vi "Batch Command.vi"() -> ()   [LabVIEW 2018]
panel:
  out "cmd sent":string
  out "test ready":string
  out "status":string
  out "mech":string
  out "state":u8
  out "S4ICS cmd":string
  out "LOG time":timestamp format="%<%H:%M:%S%3u\n%Y/%m/%d>T"
  in  "batch file":string="WPROT" caption="Batch File Name"
  in  "allin":T1={"s4icsIP"="localhost", "s4icsPort"=54165, "mech name"="", "cmd"=[], "log"=refnum} {"s4icsPort" min=1025 step=1}
  in  "stop":bool
  # "S4ICS Batch Command"
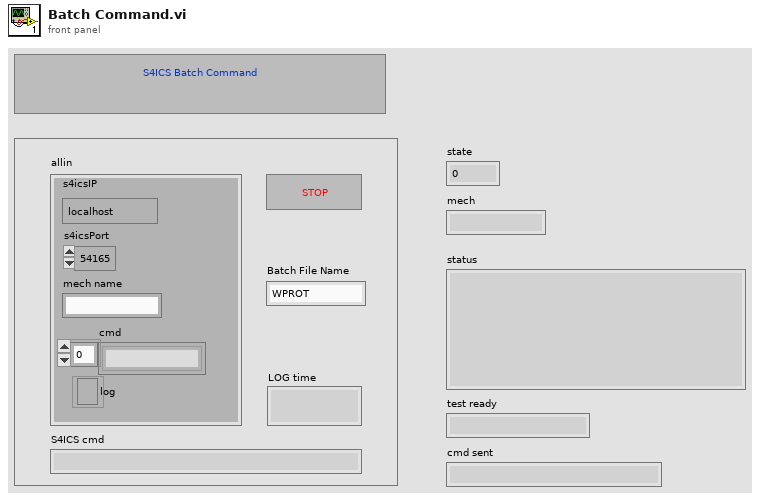
[diagram p1: front panel]
types:
  T1 = cluster{"s4icsIP":string, "s4icsPort":u16, "mech name":string, "cmd":string[], "log":refnum<file>}
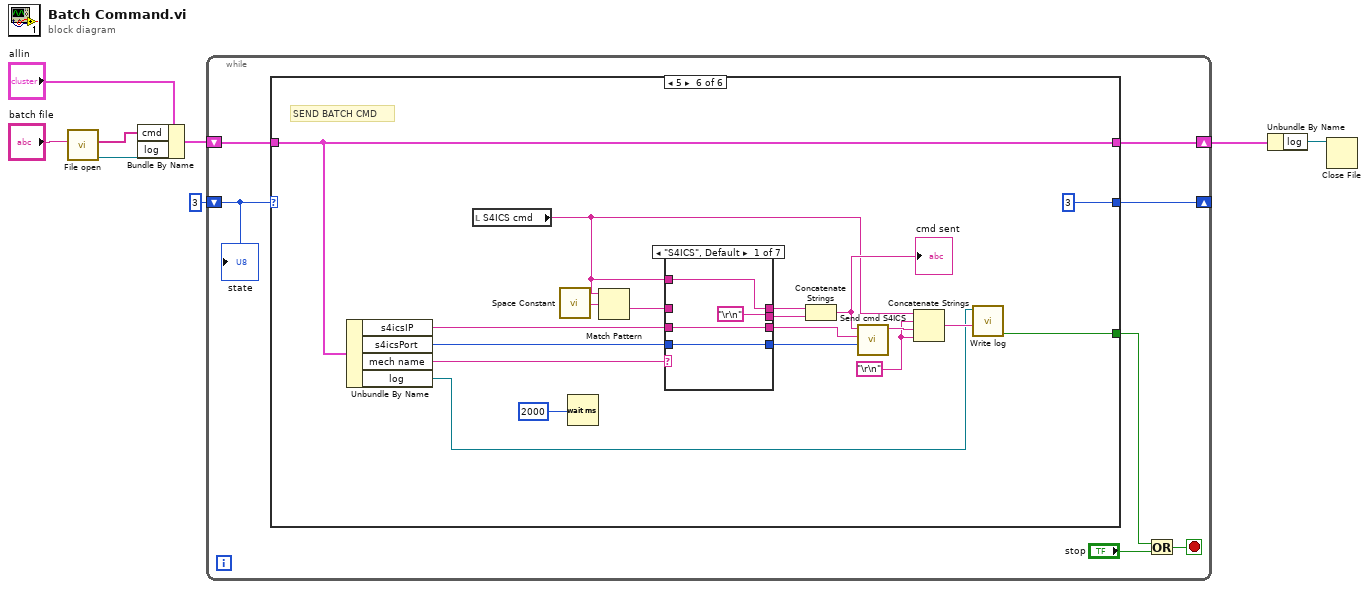
[diagram p0: block diagram]
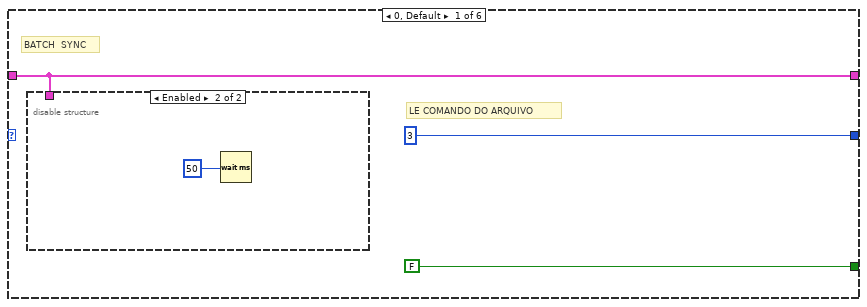
[diagram p2: hidden frame]
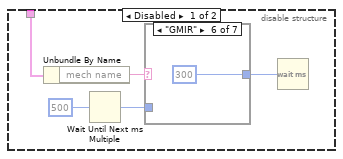
[diagram p3: hidden frame]
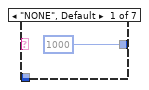
[diagram p4: hidden frame]
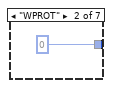
[diagram p5: hidden frame]
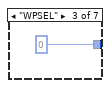
[diagram p6: hidden frame]
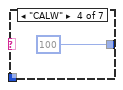
[diagram p7: hidden frame]
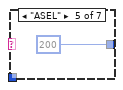
[diagram p8: hidden frame]
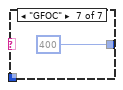
[diagram p9: hidden frame]
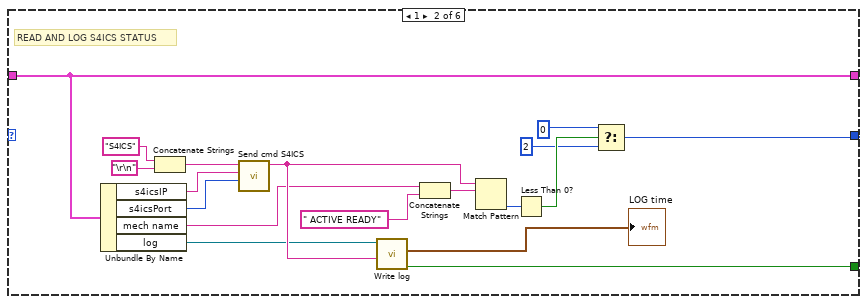
[diagram p10: hidden frame]
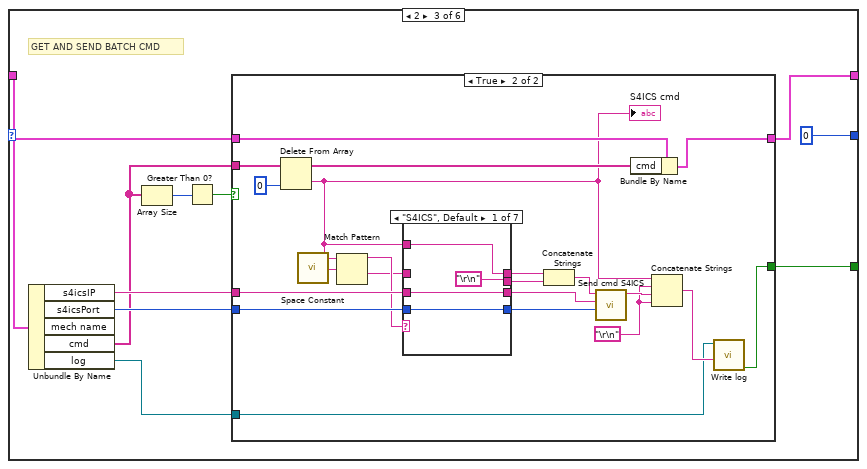
[diagram p11: hidden frame]
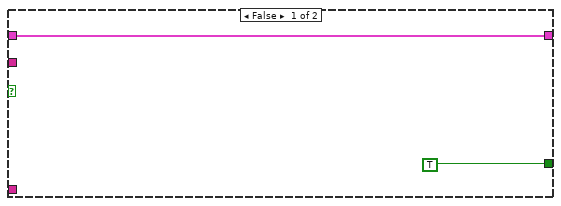
[diagram p12: hidden frame]
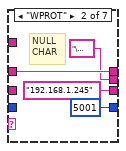
[diagram p13: hidden frame]
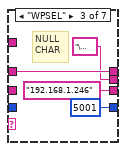
[diagram p14: hidden frame]
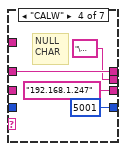
[diagram p15: hidden frame]
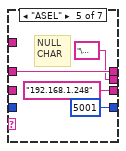
[diagram p16: hidden frame]
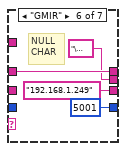
[diagram p17: hidden frame]
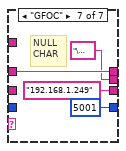
[diagram p18: hidden frame]
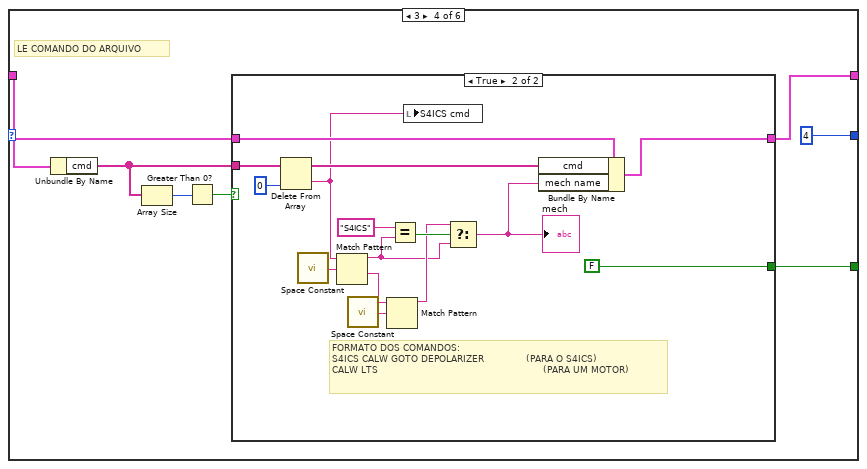
[diagram p19: hidden frame]
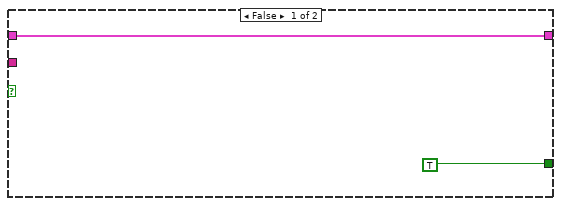
[diagram p20: hidden frame]
diagram:
  n1 = call "File open.vi"("file name"="batch file") -> ("log"=w5:refnum<file>, "cmd"=w4:string[])  [unwired: 9 in]
  n2 = Bundle By Name(cluster="allin", "cmd"=w4, "log"=w5) -> (w6:T1)
  n3 = while {
    shift-right: [w14] -> _
    shift-left: u8 3 -> [w15]
    shift-right: [w12] -> w2
    shift-left: w6 -> [w13]
    stop <- w10 stop-if-true
    n4 = case shown="5" w15 {
      tunnel: [u8 3 ("x+1") w40 u8 0 ("x+1") u8 4 ("x+1") w144 u8 3 ("x+1")] -> w14
      tunnel: w13 -> [w16 w42 w55 w115 w146 w170]
      tunnel: [w16 w42 w52 w112 w146 w170] -> w12
      tunnel: [FALSE w37 w54 w114 w141 w158] -> w9
      frame 0, Default {
        # "LE COMANDO DO ARQUIVO"
        # "BATCH  SYNC"
        n5 = disable-structure shown="Enabled" {
          disable-tunnel: w16 -> [w22 _]
          frame Disabled {
            n6 = Unbundle By Name(w22) -> ("mech name"=w21:string)
            n7 = Wait Until Next ms Multiple(millisecond multiple=u32 500) -> (millisecond timer value=w19:u32)
            n8 = case shown="\"GMIR\"" w21 {
              tunnel: [u32 1000 ("millisecond multiple") u32 0 ("millisecond multiple") u32 0 ("millisecond multiple") u32 100 ("millisecond multiple") u32 200 ("millisecond multiple") u32 300 ("millisecond multiple") u32 400 ("millisecond multiple")] -> w23
              tunnel: w19 -> [_ _ _ _ _ _ _]
              frame "NONE", Default {
              }
              frame "WPROT" {
              }
              frame "WPSEL" {
              }
              frame "CALW" {
              }
              frame "ASEL" {
              }
              frame "GMIR" {
              }
              frame "GFOC" {
              }
            }
            n9 = Wait (ms)(milliseconds to wait=w23) -> ()  [unwired: 1 out]
          }
          frame Enabled {
            n10 = Wait (ms)(milliseconds to wait=u32 50 ("millisecond multiple")) -> ()  [unwired: 1 out]
          }
        }
      }
      frame 1 {
        # "READ AND LOG S4ICS STATUS"
        n11 = Unbundle By Name(w42) -> ("s4icsIP"=w47:string, "s4icsPort"=w46:u16, "mech name"=w34:string, "log"=w36:refnum<file>)
        n12 = Concatenate Strings("S4ICS", "\r\n") -> (w45:string)
        n13 = call "Send cmd S4ICS.vi"("port"=w46, "address"=w47, "data in"=w45) -> ("data out"=w38:string)  [unwired: 7 in, 1 out]
        n14 = call "Write log.vi"("text"=w38, "log file"=w36) -> ("status"=w37:bool, "current time"=→"LOG time":timestamp)  [unwired: 8 in]
        n15 = Concatenate Strings(w34, " ACTIVE READY") -> (w35:string)
        n16 = Match Pattern(string=w38, regular expression=w35) -> (offset past match=w44:i32)  [unwired: 1 in, 3 out]
        n17 = Less Than 0?(x=w44) -> (x < 0?=w41:bool)
        n18 = Select(t=u8 0 ("f"), s=w41, f=u8 2) -> (s? t:f=w40:u8)
      }
      frame 2 {
        # "GET AND SEND BATCH CMD"
        n19 = Unbundle By Name(w55) -> ("s4icsIP"=w59:string, "s4icsPort"=w58:u16, "cmd"=w51:string[], "log"=w50:refnum<file>)  [unwired: 1 out]
        n20 = Array Size(array=w51) -> (size(s)=w57:i32)
        n21 = Greater Than 0?(x=w57) -> (x > 0?=w56:bool)
        n22 = case shown="True" w56 {
          tunnel: w59 -> [_ w72]
          tunnel: w58 -> [_ w71]
          tunnel: w51 -> [_ w82]
          tunnel: w55 -> [w61 w81]
          tunnel: [w61 w80] -> w52
          tunnel: [TRUE w76] -> w54
          tunnel: w50 -> [_ w73]
          frame False {
          }
          frame True {
            w74 = "\r\n"
            n23 = Delete From Array(array=w82, index=0) -> (deleted portion=w64:string, array with subset deleted=w77:string[])  [unwired: 1 in]
            "S4ICS cmd" <- w64
            n24 = call <vilib>:"Space Constant.vi"() -> ("String"=w67:string)
            n25 = Match Pattern(string=w64, regular expression=w67) -> (before substring=w66:string, after substring=w65:string)  [unwired: 1 in, 2 out]
            n26 = case shown="\"S4ICS\", Default" w66 {
              tunnel: w72 -> [w86 _ _ _ _ _ _]
              tunnel: w71 -> [w85 _ _ _ _ _ _]
              tunnel: [w86 "192.168.1.245" ("s4icsIP") "192.168.1.246" ("s4icsIP") "192.168.1.247" ("s4icsIP") "192.168.1.248" ("s4icsIP") "192.168.1.249" ("s4icsIP") "192.168.1.249" ("s4icsIP")] -> w70
              tunnel: [w85 u16 5001 ("s4icsPort") u16 5001 ("s4icsPort") u16 5001 ("s4icsPort") u16 5001 ("s4icsPort") u16 5001 ("s4icsPort") u16 5001 ("s4icsPort")] -> w69
              tunnel: w65 -> [_ w88 w92 w96 w100 w104 w108]
              tunnel: w64 -> [w84 _ _ _ _ _ _]
              tunnel: [w84 w88 w92 w96 w100 w104 w108] -> w63
              tunnel: ["\r\n" "\u0000" ("search string") "\u0000" ("search string") "\u0000" ("search string") "\u0000" ("search string") "\u0000" ("search string") "\u0000" ("search string")] -> w62
              frame "S4ICS", Default {
              }
              frame "WPROT" {
                # "NULL\nCHAR"
              }
              frame "WPSEL" {
                # "NULL\nCHAR"
              }
              frame "CALW" {
                # "NULL\nCHAR"
              }
              frame "ASEL" {
                # "NULL\nCHAR"
              }
              frame "GMIR" {
                # "NULL\nCHAR"
              }
              frame "GFOC" {
                # "NULL\nCHAR"
              }
            }
            n27 = Concatenate Strings(w63, w62) -> (w68:string)
            n28 = call "Send cmd S4ICS.vi"("port"=w69, "address"=w70, "data in"=w68) -> ("data out"=w79:string)  [unwired: 7 in, 1 out]
            n29 = Bundle By Name(cluster=w81, "cmd"=w77) -> (w80:T1)
            n30 = Concatenate Strings(w64, w74, w79, w74) -> (w78:string)
            n31 = call "Write log.vi"("text"=w78, "log file"=w73) -> ("status"=w76:bool)  [unwired: 8 in, 1 out]
          }
        }
      }
      frame 3 {
        # "LE COMANDO DO ARQUIVO"
        n32 = Unbundle By Name(w115) -> ("cmd"=w111:string[])
        n33 = Array Size(array=w111) -> (size(s)=w117:i32)
        n34 = Greater Than 0?(x=w117) -> (x > 0?=w116:bool)
        n35 = case shown="True" w116 {
          tunnel: w111 -> [_ w134]
          tunnel: w115 -> [w119 w133]
          tunnel: [w119 w132] -> w112
          tunnel: [TRUE FALSE] -> w114
          frame False {
          }
          frame True {
            # "FORMATO DOS COMANDOS:\nS4ICS CALW GOTO DEPOLARIZER              (PARA O S4ICS)\nCALW LTS                                                       (PARA UM MOTOR)"
            n36 = Delete From Array(array=w134, index=0) -> (deleted portion=w128:string, array with subset deleted=w131:string[])  [unwired: 1 in]
            n37 = call <vilib>:"Space Constant.vi"() -> ("String"=w129:string)
            n38 = Match Pattern(string=w128, regular expression=w129) -> (before substring=w121:string, after substring=w125:string)  [unwired: 1 in, 2 out]
            n39 = call <vilib>:"Space Constant.vi"() -> ("String"=w126:string)
            n40 = Match Pattern(string=w125, regular expression=w126) -> (before substring=w122:string)  [unwired: 1 in, 3 out]
            n41 = Equal?(x="S4ICS", y=w121) -> (x = y?=w123:bool)
            n42 = local write "S4ICS cmd"(w128) -> ()
            n43 = Select(t=w122, s=w123, f=w121) -> (s? t:f=w120:string)
            "mech" <- w120
            n44 = Bundle By Name(cluster=w133, "cmd"=w131, "mech name"=w120) -> (w132:T1)
          }
        }
      }
      frame 4 {
        # "CHECK S4ICS STATUS"
        n45 = Unbundle By Name(w146) -> ("s4icsIP"=w151:string, "s4icsPort"=w150:u16, "mech name"=w138:string, "log"=w140:refnum<file>)
        n46 = Wait (ms)(milliseconds to wait=u32 2000 ("millisecond multiple")) -> ()  [unwired: 1 out]
        n47 = Concatenate Strings("S4ICS", "\r\n") -> (w149:string)
        n48 = call "Send cmd S4ICS.vi"("port"=w150, "address"=w151, "data in"=w149) -> ("data out"=w142:string)  [unwired: 7 in, 1 out]
        "status" <- w142
        n49 = call "Write log.vi"("text"=w142, "log file"=w140) -> ("status"=w141:bool, "current time"=w136:timestamp)  [unwired: 8 in]
        n50 = Concatenate Strings(w138, " ACTIVE READY") -> (w139:string)
        "test ready" <- w139
        n51 = local write "LOG time"(w136) -> ()
        n52 = Match Pattern(string=w142, regular expression=w139) -> (offset past match=w148:i32)  [unwired: 1 in, 3 out]
        n53 = Less Than 0?(x=w148) -> (x < 0?=w145:bool)
        n54 = Select(t=u8 4 ("f"), s=w145, f=u8 5) -> (s? t:f=w144:u8)
      }
      frame 5 {
        w166 = "\r\n"
        # "SEND BATCH CMD"
        n55 = Unbundle By Name(w170) -> ("s4icsIP"=w172:string, "s4icsPort"=w171:u16, "mech name"=w155:string, "log"=w156:refnum<file>)
        n56 = local read "S4ICS cmd"() -> (w157:string)
        n57 = call <vilib>:"Space Constant.vi"() -> ("String"=w162:string)
        n58 = Wait (ms)(milliseconds to wait=u32 2000 ("millisecond multiple")) -> ()  [unwired: 1 out]
        n59 = Match Pattern(string=w157, regular expression=w162) -> (after substring=w161:string)  [unwired: 1 in, 3 out]
        n60 = case shown="\"S4ICS\", Default" w155 {
          tunnel: w172 -> [w176 _ _ _ _ _ _]
          tunnel: w171 -> [w175 _ _ _ _ _ _]
          tunnel: [w176 "192.168.1.245" ("s4icsIP") "192.168.1.246" ("s4icsIP") "192.168.1.247" ("s4icsIP") "192.168.1.248" ("s4icsIP") "192.168.1.249" ("s4icsIP") "192.168.1.249" ("s4icsIP")] -> w165
          tunnel: [w175 u16 5001 ("s4icsPort") u16 5001 ("s4icsPort") u16 5001 ("s4icsPort") u16 5001 ("s4icsPort") u16 5001 ("s4icsPort") u16 5001 ("s4icsPort")] -> w164
          tunnel: w161 -> [_ w178 w182 w186 w190 w194 w198]
          tunnel: w157 -> [w174 _ _ _ _ _ _]
          tunnel: [w174 w178 w182 w186 w190 w194 w198] -> w160
          tunnel: ["\r\n" "\u0000" ("search string") "\u0000" ("search string") "\u0000" ("search string") "\u0000" ("search string") "\u0000" ("search string") "\u0000" ("search string")] -> w159
          frame "S4ICS", Default {
          }
          frame "WPROT" {
            # "NULL\nCHAR"
          }
          frame "WPSEL" {
            # "NULL\nCHAR"
          }
          frame "CALW" {
            # "NULL\nCHAR"
          }
          frame "ASEL" {
            # "NULL\nCHAR"
          }
          frame "GMIR" {
            # "NULL\nCHAR"
          }
          frame "GFOC" {
            # "NULL\nCHAR"
          }
        }
        n61 = Concatenate Strings(w160, w159) -> (w163:string)
        "cmd sent" <- w163
        n62 = call "Send cmd S4ICS.vi"("port"=w164, "address"=w165, "data in"=w163) -> ("data out"=w168:string)  [unwired: 7 in, 1 out]
        n63 = Concatenate Strings(w157, w166, w168, w166) -> (w167:string)
        n64 = call "Write log.vi"("text"=w167, "log file"=w156) -> ("status"=w158:bool)  [unwired: 8 in, 1 out]
      }
    }
    n65 = Or(x=w9, y="stop") -> (x .or. y?=w10:bool)
    "state" <- w15
  }
  n66 = Unbundle By Name(w2) -> ("log"=w1:refnum<file>)
  n67 = Close File(refnum=w1) -> ()  [unwired: 1 in, 2 out]
